vi "PTScanner.reset.vi"(0 "i ref in":refnum<vi>, 5 "error in (no error)":errorcluster) -> (14 "i ref out":refnum<vi>, 19 "error out":errorcluster)   [LabVIEW 2014, in "PTScanner.lvlib"]
uses:
  PTScanner.lvlib
  CSlibraries-extern/DimLVEvent/LVDimInterface/LVDimInterface.lvlib
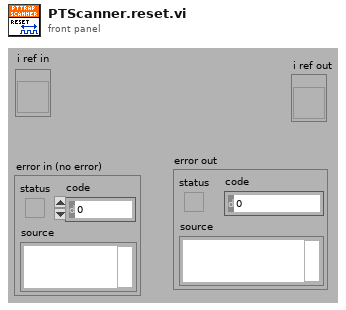
[diagram p1: front panel]
types:
  T1 = typedef "PTScanner.lvlib/PTScanner.i attribute.ctl" = cluster{"Object cmds":T2[], "Steps":cluster{"Finished":bool, "cmd setup":T3[]}[], "curStep":i32, "DIM IDs":cluster{"AllFinished":i32, "Finished":i32, "curStep":i32, "nofSteps":i32, "NomValues":i32[], "1D-Min":i32, "1D-Max":i32, "Dimensions":i32, "MaxDimensions":i32, "ScanedDeviceNames":i32[]}, "All Finished":bool, "DIMs in use":string[], "Running":bool, "Scan Delay":u32, "loop":bool, "Paused":bool, "Formed":bool}
  T2 = typedef "PTScanner.lvlib/PTScanner.obj parameters.ctl" = cluster{"object":string, "DIM address":string, "method":string, "data descriptor":string, "method parameters":cluster{"Name":string, "Descr":string, "Value":string, "Value?":bool}[], "Call Mode":enum16{"Simple DIM", "Synchronous"}, "actValue":dbl, "Centroid":dbl, "Minus Delta":dbl, "Plus Delta":dbl, "increment":dbl, "DIM Status":cluster{"no link":bool, "quality":i32, "Time Stamp":timestamp}, "range":dbl, "DIMChannelIndex":i32}
  T3 = typedef "PTScanner.lvlib/PTScanner.step obj parameters.ctl" = cluster{"obj index":i32, "nomValue":dbl, "fulfilled":bool}
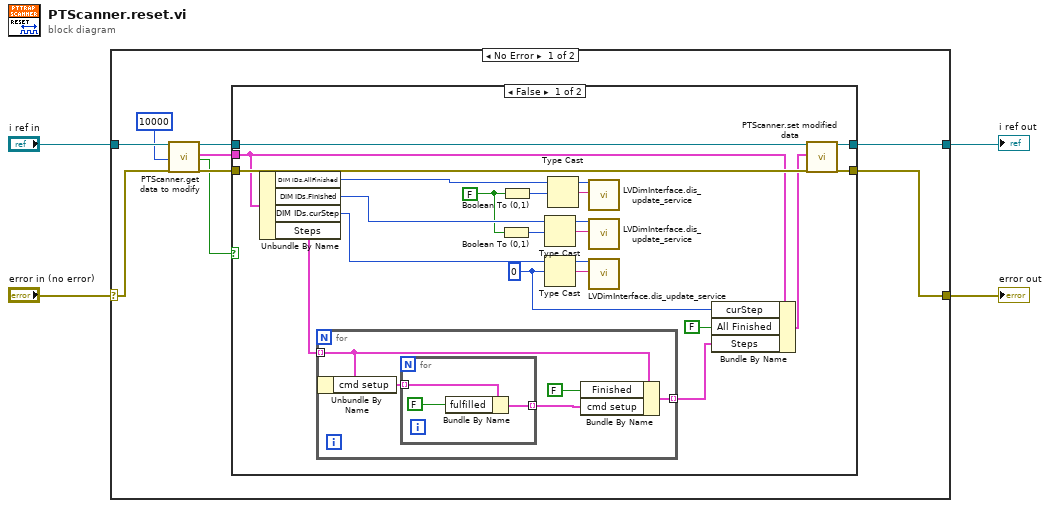
[diagram p0: block diagram]
diagram:
  n1 = case shown="No Error" "error in (no error)" {
    selector: "error in (no error)" -> [w8 w43]
    tunnel: "i ref in" -> [w9 w44]
    tunnel: [w5 w43] -> w3
    tunnel: [w6 w44] -> w2
    frame No Error {
      n2 = call "PTScanner.get data to modify.vi"("i ref in"=w9, "ms timeout (10000)"=10000, "error in (no error)"=w8) -> ("i ref out"=w13:refnum<vi>, "i attribute"=w10:T1, "timed out"=w11:bool, "error out"=w12:errorcluster)  [unwired: 13 in]
      n3 = case shown="False" w11 {
        tunnel: w13 -> [w32 w42]
        tunnel: [w28 w42] -> w6
        tunnel: [w27 w41] -> w5
        tunnel: w12 -> [w31 w41]
        tunnel: w10 -> [w30 _]
        frame False {
          w14 = 0
          w22 = FALSE
          n4 = Unbundle By Name(w30) -> ("DIM IDs.AllFinished"=w26:i32, "DIM IDs.Finished"=w24:i32, "DIM IDs.curStep"=w16:i32, "Steps"=w17:cluster{"Finished":bool, "cmd setup":T3[]}[])
          n5 = for {
            tunnel: w17 -> [w35] mode=indexing
            tunnel: [w36] -> w18 mode=indexing
            n6 = Unbundle By Name(w35) -> ("cmd setup"=w34:T3[])
            n7 = for {
              tunnel: w34 -> [w40] mode=indexing
              tunnel: [w38] -> w33 mode=indexing
              n8 = Bundle By Name(cluster=w40, "fulfilled"=FALSE) -> (w38:T3)
            }
            n9 = Bundle By Name(cluster=w35, "Finished"=FALSE, "cmd setup"=w33) -> (w36:cluster{"Finished":bool, "cmd setup":T3[]})
          }
          n10 = Boolean To (0,1)(Boolean=w22) -> (0, 1=w20:i16)
          n11 = Boolean To (0,1)(Boolean=w22) -> (0, 1=w21:i16)
          n12 = Type Cast(x=w20) -> (*(type *) &x=w23:string)  [unwired: 1 in]
          n13 = Type Cast(x=w14) -> (*(type *) &x=w15:string)  [unwired: 1 in]
          n14 = Type Cast(x=w21) -> (*(type *) &x=w25:string)  [unwired: 1 in]
          n15 = call "LVDimInterface.dis_update_service.vi"("my_serviceID"=w26, "data"=w25) -> ()  [unwired: 15 in, 3 out]
          n16 = call "LVDimInterface.dis_update_service.vi"("my_serviceID"=w24, "data"=w23) -> ()  [unwired: 15 in, 3 out]
          n17 = call "LVDimInterface.dis_update_service.vi"("my_serviceID"=w16, "data"=w15) -> ()  [unwired: 15 in, 3 out]
          n18 = Bundle By Name(cluster=w30, "curStep"=w14, "All Finished"=FALSE, "Steps"=w18) -> (w29:T1)
          n19 = call "PTScanner.set modified data.vi"("i ref in"=w32, "CLASS.i attribute"=w29, "error in (no error)"=w31) -> ("i ref out"=w28:refnum<vi>, "error out"=w27:errorcluster)  [unwired: 15 in]
        }
        frame True {
        }
      }
    }
    frame Error {
    }
  }
  "error out" <- w3
  "i ref out" <- w2
